vi "constant stuff.vi"() -> ()   [LabVIEW 2015]
uses:
  <vilib>/Analysis/baseanly.llb/Mean (DBL).vi
  <vilib>/gmath/SpecialFunctions.llb/Factorial.vi
  <vilib>/Utility/file.llb/Read Delimited Spreadsheet (DBL).vi
  <vilib>/imath/engines/lvmath2/RunTimeEngine/Managers/WorkSpace/UID Generator.vi
  <vilib>/imath/engines/lvmath2/RunTimeEngine/ArithmeticOperatorToken/NIMS_ArithmeticOperator_power(S).vi
  <instcachedir>/0/NIMS_ArithmeticOperator_power(S)_DFB67823F1414E5097C86E39787D8CA8.lvgen/NIMS_ArithmeticOperator_power(S)_DFB67823F1414E5097C86E39787D8CA8_014.vi
  <vilib>/imath/engines/lvmath2/RunTimeEngine/RunTimeType/NIMS_RunTimeType_From StrictType (excl LVString).vi
  <instcachedir>/0/NIMS_RunTimeType_From StrictType (excl LVString)_EB1C38A9BC5048DA9ABDA8F781E54D21.lvgen/NIMS_RunTimeType_From StrictType (excl LVString)_EB1C38A9BC5048DA9ABDA8F781E54D21_000.vi
  <vilib>/imathl/engines/lvmath/Functions/Error Handling/Create Error.vi
  <vilib>/imath/engines/lvmath2/RunTimeEngine/LocalVariableDefStatement/MC_LocalVariableDefStatement_Display.vi
  <vilib>/imath/engines/lvmath2/RunTimeEngine/Managers/SymbolTable/Clear UID.vi
  <vilib>/imath/engines/lvmath2/RunTimeEngine/NodeEndStatement/NIMS_NodeEndStatement_Output.vi
  <instcachedir>/0/NIMS_NodeEndStatement_Output_53EC0D466D134D7ABD903AC30B43404B.lvgen/NIMS_NodeEndStatement_Output_53EC0D466D134D7ABD903AC30B43404B_009.vi
  <vilib>/imath/engines/lvmath2/RunTimeEngine/ErrorHandling/NIMS_Finalize Error.vi
  <vilib>/Analysis/NI_AALBase.lvlib
  <vilib>/gmath/NI_Gmath.lvlib
  <vilib>/imath/engines/lvmath2/RunTimeEngine/Managers/SymbolTable/NIMS_WorkSpace.lvlib
panel:
  out "XY Graph":cluster{"X Values":dbl[], dbl[]}[](graph)=[{"X Values"=[37.45, 38.35, 39.25, 40.15, 41.05, 41.95, 42.85, 43.75, 44.65, 45.55, 46.45, 47.35, 48.25, 49.15, 50.05, 50.95, 51.85, 52.75, 53.65, 54.55, 55.45, 56.35, 57.25, 58.15, 59.05, 59.95, 60.85, 61.75, 62.65, 63.55, 64.45, 65.35, 66.25, 67.15, 68.05, 68.95, 69.85, 70.75, 71.65, 72.55], [1.0, 1.0, 1.0, 4.0, 2.0, 3.0, 2.0, 1.0, 6.0, 0.0, 7.0, 4.0, 5.0, 4.0, 3.0, 8.0, 5.0, 2.0, 6.0, 0.0, 7.0, 6.0, 8.0, 4.0, 4.0, 3.0, 4.0, 5.0, 3.0, 0.0, 3.0, 3.0, 1.0, 0.0, 1.0, 1.0, 0.0, 0.0, 0.0, 1.0]}, {"X Values"=[57.0, 51.0, 48.0, 55.0, 49.0, 64.0, 62.0, 64.0, 58.0, 56.0, 59.0, 54.0, 49.0, 51.0, 50.0, 46.0, 40.0, 73.0, 54.0, 51.0, 61.0, 45.0, 59.0, 39.0, 57.0, 54.0, 62.0, 45.0, 42.0, 41.0, 55.0, 46.0, 60.0, 52.0, 51.0, 59.0, 55.0, 61.0, 56.0, 54.0, 65.0, 43.0, 58.0, 56.0, 48.0, 56.0, 50.0, 62.0, 55.0, 61.0, 51.0, 56.0, 66.0, 62.0, 57.0, 53.0, 49.0, 42.0, 63.0, 43.0, 37.0, 51.0, 69.0, 45.0, 52.0, 57.0, 62.0, 44.0, 60.0, 55.0, 40.0, 53.0, 57.0, 56.0, 48.0, 47.0, 40.0, 45.0, 47.0, 58.0, 47.0, 50.0, 48.0, 65.0, 51.0, 54.0, 45.0, 63.0, 51.0, 55.0, 47.0, 41.0, 38.0, 40.0, 42.0, 48.0, 55.0, 61.0, 64.0, 57.0, 57.0, 59.0, 52.0, 52.0, 46.0, 58.0, 49.0, 65.0, 46.0, 54.0, 60.0, 63.0, 52.0, 45.0, 46.0, 46.0, 57.0, 68.0, 46.0], [6.62370115716595, 7.808076463958851, 6.55318923790551, 7.526825950044112, 7.088143461408068, 2.4851837988270105, 3.567198674571133, 2.4851837988270105, 6.052692436720666, 7.123603131291613, 5.4371643923082935, 7.810857117970233, 7.088143461408068, 7.808076463958851, 7.513432069092408, 5.263081139449972, 1.6014355772586812, 0.2327766943658955, 7.810857117970233, 7.808076463958851, 4.172949392894612, 4.567957215371631, 5.4371643923082935, 1.208630624346163, 6.62370115716595, 7.810857117970233, 3.567198674571133, 4.567957215371631, 2.6123301605804836, 2.070148429139232, 7.526825950044112, 5.263081139449972, 4.802828546539037, 7.95823178057352, 7.808076463958851, 5.4371643923082935, 7.526825950044112, 4.172949392894612, 7.123603131291613, 7.810857117970233, 2.026380635966658, 3.2198488025759753, 6.052692436720666, 7.123603131291613, 6.55318923790551, 7.123603131291613, 7.513432069092408, 3.567198674571133, 7.526825950044112, 4.172949392894612, 7.808076463958851, 7.123603131291613, 1.627245056155012, 3.567198674571133, 6.62370115716595, 7.958231780573369, 7.088143461408068, 2.6123301605804836, 3.000976662734474, 3.2198488025759753, 0.637661297714856, 7.808076463958851, 0.7706332856980754, 4.567957215371631, 7.95823178057352, 6.62370115716595, 3.567198674571133, 3.878454239466442, 4.802828546539037, 7.526825950044112, 1.6014355772586812, 7.958231780573369, 6.62370115716595, 7.123603131291613, 6.55318923790551, 5.934963838103046, 1.6014355772586812, 4.567957215371631, 5.934963838103046, 6.052692436720666, 5.934963838103046, 7.513432069092408, 6.55318923790551, 2.026380635966658, 7.808076463958851, 7.810857117970233, 4.567957215371631, 3.000976662734474, 7.808076463958851, 7.526825950044112, 5.934963838103046, 2.070148429139232, 0.8893697047075455, 1.6014355772586812, 2.6123301605804836, 6.55318923790551, 7.526825950044112, 4.172949392894612, 2.4851837988270105, 6.62370115716595, 6.62370115716595, 5.4371643923082935, 7.95823178057352, 7.95823178057352, 5.263081139449972, 6.052692436720666, 7.088143461408068, 2.026380635966658, 5.263081139449972, 7.810857117970233, 4.802828546539037, 3.000976662734474, 7.95823178057352, 4.567957215371631, 5.263081139449972, 5.263081139449972, 6.62370115716595, 1.0032772964748717, 5.263081139449972]}]
  in  "Numeric":i32=119
  in  "file path (dialog if empty)":path
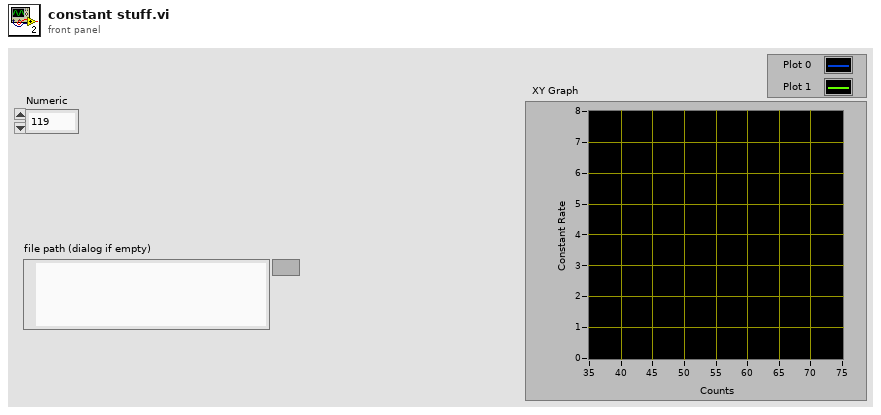
[diagram p1: front panel]
types:
  T1 = cluster{"X Values":dbl[], "Histogram: h(x)":i32[]}
  T2 = cluster{"all rows":dbl[], "Histogram: h(x)":cdb[]}[]
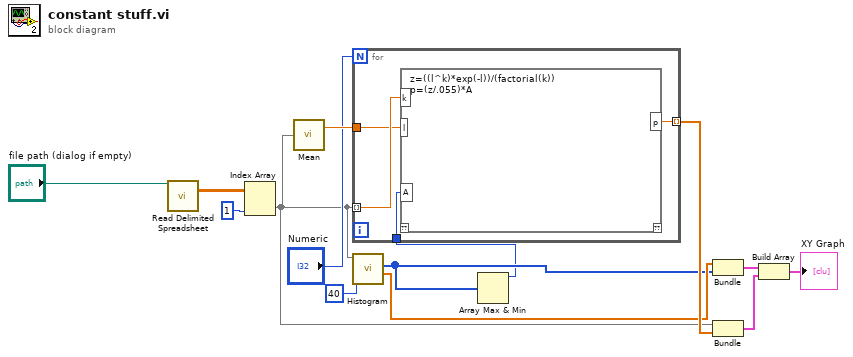
[diagram p0: block diagram]
diagram:
  n1 = call-poly <vilib>:"Read Delimited Spreadsheet.vi"("file path (dialog if empty)"="file path (dialog if empty)") -> ("all rows"=w12:dbl[][])  [unwired: 9 in, 5 out]
  n2 = Index Array(array=w12, index (col)=1 ("disabled index (col)")) -> (element=w4:dbl[])  [unwired: 1 in]
  n3 = call-poly <vilib>:"Mean.vi"("X"=w4) -> ("mean"=w11:dbl)  [unwired: 1 out]
  n4 = call <vilib>:"Histogram.vi"("intervals"=40, "X"=w4) -> ("X Values"=w5:dbl[], "Histogram: h(x)"=w3:i32[])  [unwired: 6 in, 2 out]
  n5 = Array Max & Min(array=w3) -> (max value=w2:i32)  [unwired: 3 out]
  n6 = for {
    N: "Numeric" -> [_]
    tunnel: w4 -> [w18] mode=indexing
    tunnel: [w17] -> w10 mode=indexing
    tunnel: w11 -> [w16]
    tunnel: w2 -> [w15]
    n7 = mathscript code="z=((l^k)*exp(-l))/(factorial(k))\np=(z/.055)*A"("k"=w18, "l"=w16, "A"=w15) -> ("p"=w17:cdb)  [unwired: 1 in, 1 out]
  }
  n8 = Bundle("X Values"=w5, "Histogram: h(x)"=w3) -> (w8:T1)  [unwired: 1 in]
  n9 = Bundle("all rows"=w4, w10) -> (w6:cluster{"all rows":dbl[], cdb[]})  [unwired: 1 in]
  n10 = Build Array(w8, w6) -> (→"XY Graph":T2)
